vi "F1Machine.vi"() -> ()   [LabVIEW 2011]
doc: "使用该模板构建标准状态机设计模式。各状态执行代码并决定转移状态。将该设计模式与根据用户动作响应而执行代码的用户界面事件处理器模式相比较。同时将该设计模式与队列消息处理模式（各消息处理代码可排队0个或多个新消息）。"
uses:
  F1State.ctl
  API/API DYM.lvlib
panel:
  in  "停止":bool
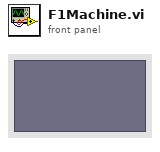
[diagram p1: front panel]
types:
  T1 = typedef "F1State.ctl" = enum16{"Initialize", "Stop", "推送物料", "推料气缸复位", "物件到位检测-光电漫射", "物体属性检测-电涡流", "分拣物体", "不分拣物体", "物件到位检测-电容式接近开关", "气缸机构运动", "气缸机构复位"}
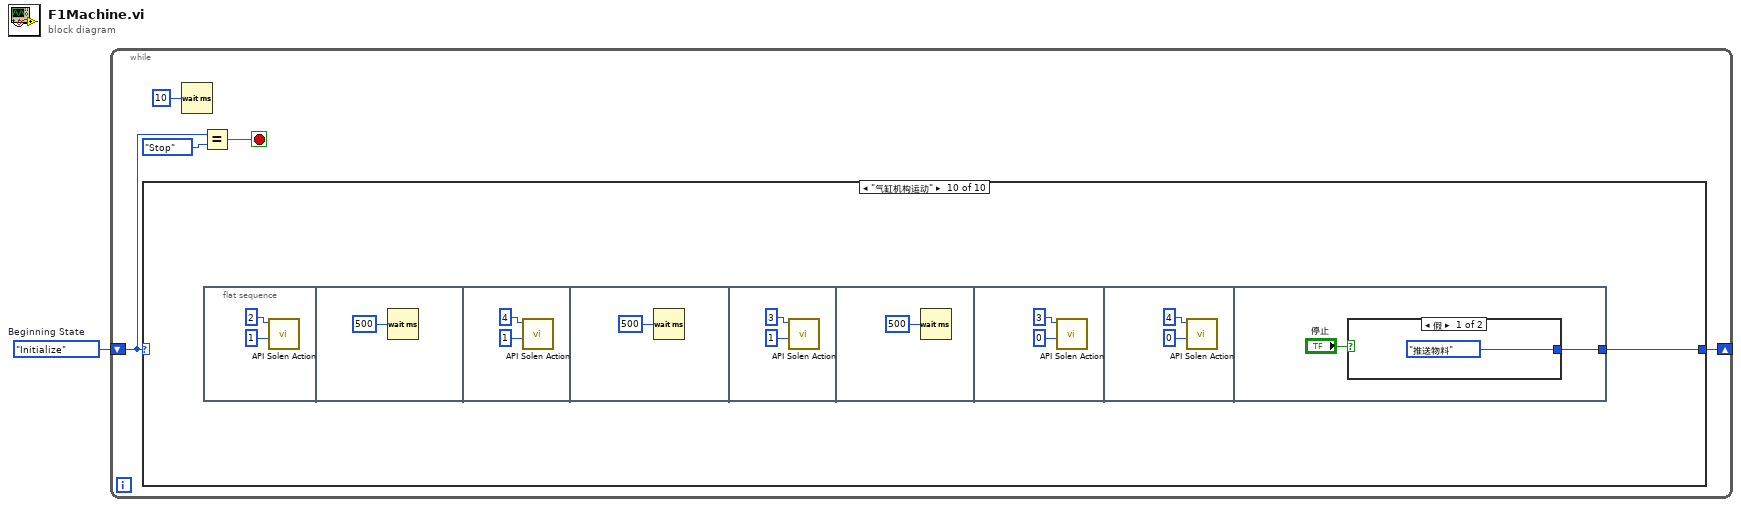
[diagram p0: block diagram]
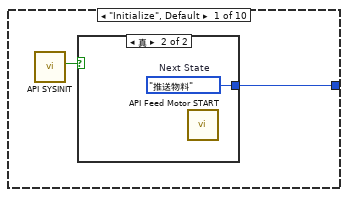
[diagram p2: hidden frame]
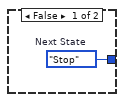
[diagram p3: hidden frame]
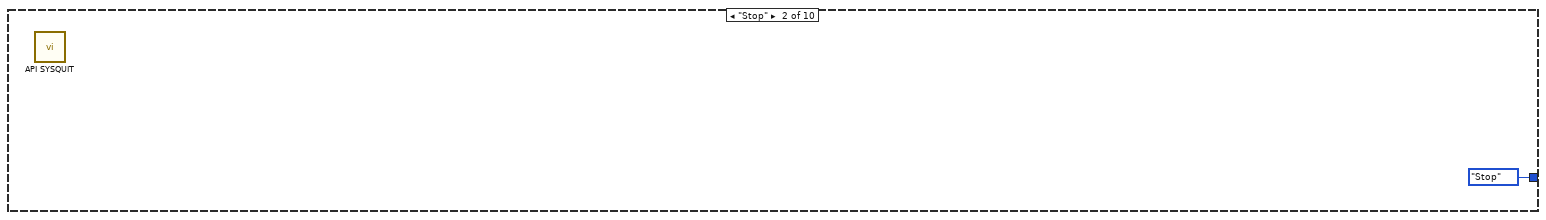
[diagram p4: hidden frame]
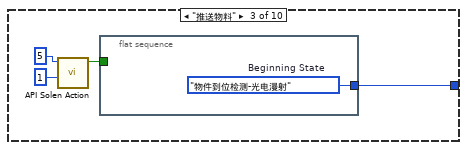
[diagram p5: hidden frame]
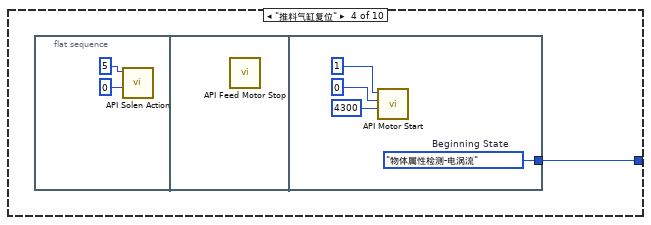
[diagram p6: hidden frame]
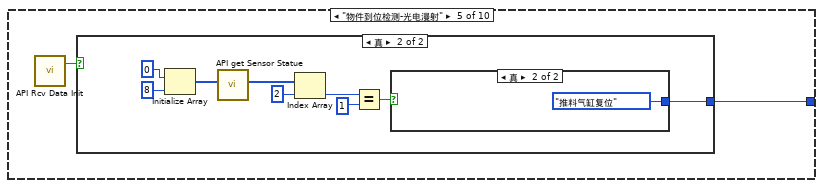
[diagram p7: hidden frame]
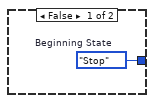
[diagram p8: hidden frame]
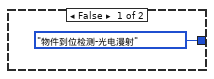
[diagram p9: hidden frame]
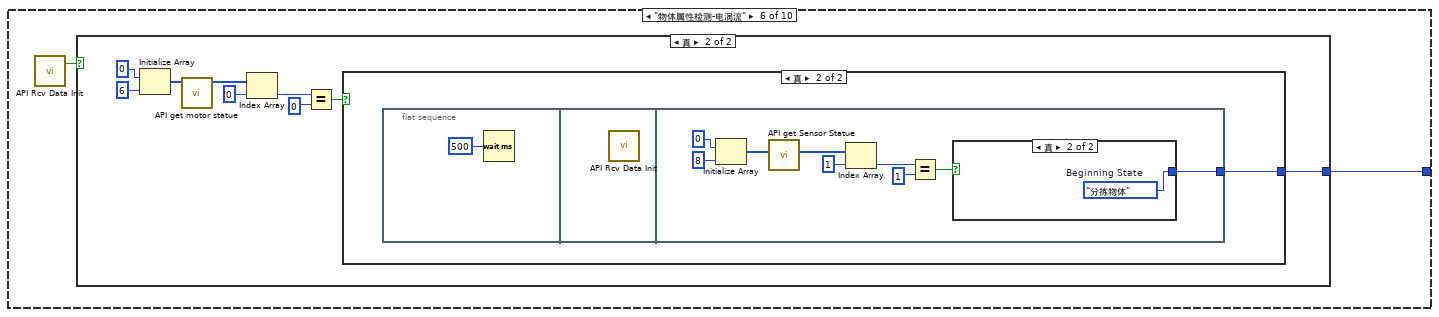
[diagram p10: hidden frame]
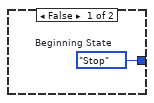
[diagram p11: hidden frame]
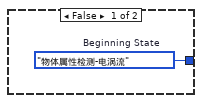
[diagram p12: hidden frame]
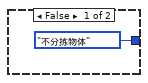
[diagram p13: hidden frame]
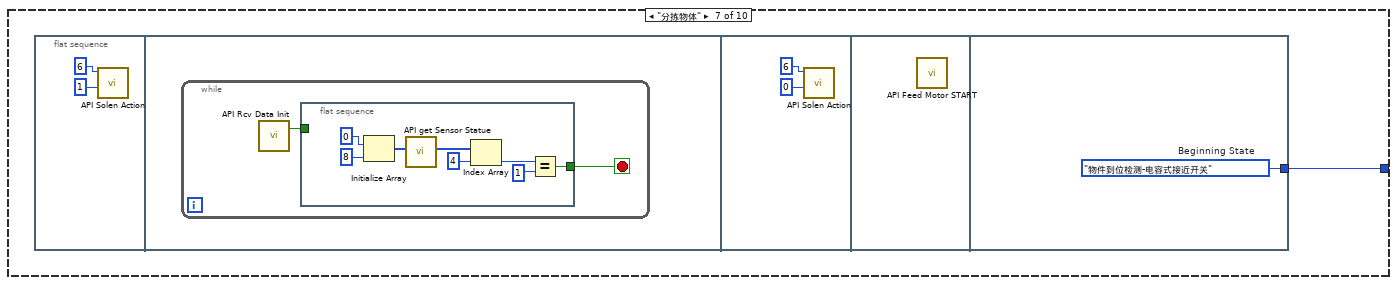
[diagram p14: hidden frame]
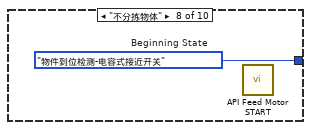
[diagram p15: hidden frame]
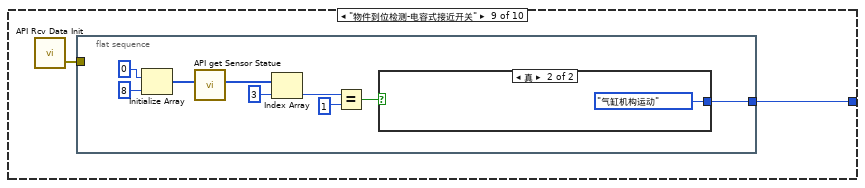
[diagram p16: hidden frame]
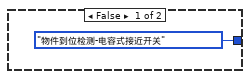
[diagram p17: hidden frame]
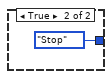
[diagram p18: hidden frame]
diagram:
  w1 = F1State."Initialize"  # Beginning State
  n1 = while {
    shift-right: [w3] -> _
    shift-left: w1 -> [w4]
    stop <- w6 stop-if-true
    n2 = case shown="\"气缸机构运动\"" w4 {
      tunnel: [w7 F1State."Stop" ("Next State") w12 w17 w24 w38 w64 w80 w81 w94] -> w3
      frame "Initialize", Default {
        n3 = call "API SYSINIT.vi"() -> ("SYSINIT return value"=w8:bool)  [unwired: 11 in]
        n4 = case shown="真" w8 {
          tunnel: [w9 w10] -> w7
          frame False {
            w9 = F1State."Stop"  # Next State
          }
          frame True {
            w10 = F1State."推送物料"  # Next State
            n5 = call "API Feed Motor START.vi"() -> ()  [unwired: 11 in, 1 out]
          }
        }
      }
      frame "Stop" {
        n6 = call "API SYSQUIT.vi"() -> ()  [unwired: 12 in]
      }
      frame "推送物料" {
        n7 = call "API Solen Action.vi"("statue"=1, "solenNum"=5) -> ("solenaction return value"=w13:bool)  [unwired: 9 in]
        n8 = flat-sequence {
          tunnel: w13 -> [_]
          tunnel: [w16] -> w12
          frame #0 {
            w16 = F1State."物件到位检测-光电漫射"  # Beginning State
          }
        }
      }
      frame "推料气缸复位" {
        n9 = flat-sequence {
          tunnel: [w20] -> w17
          frame #0 {
            n10 = call "API Solen Action.vi"("statue"=0, "solenNum"=5) -> ()  [unwired: 9 in, 1 out]
          }
          frame #1 {
            n11 = call "API Feed Motor Stop.vi"() -> ()  [unwired: 11 in, 1 out]
          }
          frame #2 {
            w20 = F1State."物体属性检测-电涡流"  # Beginning State
            n12 = call "API Motor Start.vi"("stepNum"=4300, "direction"=0, "motorNum"=1) -> ()  [unwired: 8 in, 1 out]
          }
        }
      }
      frame "物件到位检测-光电漫射" {
        n13 = call "API Rcv Data Init.vi"() -> ("RTV"=w25:bool)  [unwired: 2 in, 1 out]
        n14 = case shown="真" w25 {
          tunnel: [w26 w27] -> w24
          frame False {
            w26 = F1State."Stop"  # Beginning State
          }
          frame True {
            n15 = Initialize Array(0 ("元素"), 8 ("维数大小")) -> (w33:i32[])
            n16 = call "API get Sensor Statue.vi"("array input"=w33) -> ("array output"=w32:i32[])  [unwired: 9 in, 1 out]
            n17 = Index Array(array=w32, index=2 ("索引")) -> (element=w30:i32)
            n18 = Equal?(x=w30, y=1) -> (x = y?=w28:bool)
            n19 = case shown="真" w28 {
              tunnel: [F1State."物件到位检测-光电漫射" ("Beginning State") F1State."推料气缸复位" ("Beginning State")] -> w27
              frame False {
              }
              frame True {
              }
            }
          }
        }
      }
      frame "物体属性检测-电涡流" {
        n20 = call "API Rcv Data Init.vi"() -> ("RTV"=w39:bool)  [unwired: 2 in, 1 out]
        n21 = case shown="真" w39 {
          tunnel: [w40 w41] -> w38
          frame False {
            w40 = F1State."Stop"  # Beginning State
          }
          frame True {
            n22 = Initialize Array(0 ("元素"), 6 ("维数大小")) -> (w47:i32[])
            n23 = call "API get motor statue.vi"("motor statue array input"=w47) -> ("motor statue array output"=w46:i32[])  [unwired: 9 in, 1 out]
            n24 = Index Array(array=w46, index=0 ("索引")) -> (element=w44:i32)
            n25 = Equal?(x=w44, y=0) -> (x = y?=w42:bool)
            n26 = case shown="真" w42 {
              tunnel: [w50 w51] -> w41
              frame False {
                w50 = F1State."物体属性检测-电涡流"  # Beginning State
              }
              frame True {
                n27 = flat-sequence {
                  tunnel: [w53] -> w51
                  frame #0 {
                    n28 = Wait (ms)(milliseconds to wait=u32 500) -> ()  [unwired: 1 out]
                  }
                  frame #1 {
                    n29 = call "API Rcv Data Init.vi"() -> ()  [unwired: 2 in, 2 out]
                  }
                  frame #2 {
                    n30 = Initialize Array(0 ("元素"), 8 ("维数大小")) -> (w59:i32[])
                    n31 = call "API get Sensor Statue.vi"("array input"=w59) -> ("array output"=w58:i32[])  [unwired: 9 in, 1 out]
                    n32 = Index Array(array=w58, index=1 ("索引")) -> (element=w55:i32)
                    n33 = Equal?(x=w55, y=1) -> (x = y?=w54:bool)
                    n34 = case shown="真" w54 {
                      tunnel: [F1State."不分拣物体" ("Beginning State") w63] -> w53
                      frame False {
                      }
                      frame True {
                        w63 = F1State."分拣物体"  # Beginning State
                      }
                    }
                  }
                }
              }
            }
          }
        }
      }
      frame "分拣物体" {
        n35 = flat-sequence {
          tunnel: [w79] -> w64
          frame #0 {
            n36 = call "API Solen Action.vi"("statue"=1, "solenNum"=6) -> ()  [unwired: 9 in, 1 out]
          }
          frame #1 {
            n37 = while {
              stop <- w68 stop-if-true
              n38 = call "API Rcv Data Init.vi"() -> ("RTV"=w67:bool)  [unwired: 2 in, 1 out]
              n39 = flat-sequence {
                tunnel: [w69] -> w68
                tunnel: w67 -> [_]
                frame #0 {
                  n40 = Initialize Array(0 ("元素"), 8 ("维数大小")) -> (w74:i32[])
                  n41 = call "API get Sensor Statue.vi"("array input"=w74) -> ("array output"=w73:i32[])  [unwired: 9 in, 1 out]
                  n42 = Index Array(array=w73, index=4 ("索引")) -> (element=w71:i32)
                  n43 = Equal?(x=w71, y=1) -> (x = y?=w69:bool)
                }
              }
            }
          }
          frame #2 {
            n44 = call "API Solen Action.vi"("statue"=0, "solenNum"=6) -> ()  [unwired: 9 in, 1 out]
          }
          frame #3 {
            n45 = call "API Feed Motor START.vi"() -> ()  [unwired: 11 in, 1 out]
          }
          frame #4 {
            w79 = F1State."物件到位检测-电容式接近开关"  # Beginning State
          }
        }
      }
      frame "不分拣物体" {
        w80 = F1State."物件到位检测-电容式接近开关"  # Beginning State
        n46 = call "API Feed Motor START.vi"() -> ()  [unwired: 11 in, 1 out]
      }
      frame "物件到位检测-电容式接近开关" {
        n47 = call "API Rcv Data Init.vi"() -> ("错误输出"=w82:errorcluster)  [unwired: 2 in, 1 out]
        n48 = flat-sequence {
          tunnel: w82 -> [_]
          tunnel: [w83] -> w81
          frame #0 {
            n49 = Initialize Array(0 ("元素"), 8 ("维数大小")) -> (w89:i32[])
            n50 = call "API get Sensor Statue.vi"("array input"=w89) -> ("array output"=w88:i32[])  [unwired: 9 in, 1 out]
            n51 = Index Array(array=w88, index=3 ("索引")) -> (element=w86:i32)
            n52 = Equal?(x=w86, y=1) -> (x = y?=w84:bool)
            n53 = case shown="真" w84 {
              tunnel: [F1State."物件到位检测-电容式接近开关" ("Beginning State") F1State."气缸机构运动" ("Beginning State")] -> w83
              frame False {
              }
              frame True {
              }
            }
          }
        }
      }
      frame "气缸机构运动" {
        n54 = flat-sequence {
          tunnel: [w108] -> w94
          frame #0 {
            n55 = call "API Solen Action.vi"("statue"=1, "solenNum"=2) -> ()  [unwired: 9 in, 1 out]
          }
          frame #1 {
            n56 = Wait (ms)(milliseconds to wait=u32 500) -> ()  [unwired: 1 out]
          }
          frame #2 {
            n57 = call "API Solen Action.vi"("statue"=1, "solenNum"=4) -> ()  [unwired: 9 in, 1 out]
          }
          frame #3 {
            n58 = Wait (ms)(milliseconds to wait=u32 500) -> ()  [unwired: 1 out]
          }
          frame #4 {
            n59 = call "API Solen Action.vi"("statue"=1, "solenNum"=3) -> ()  [unwired: 9 in, 1 out]
          }
          frame #5 {
            n60 = Wait (ms)(milliseconds to wait=u32 500) -> ()  [unwired: 1 out]
          }
          frame #6 {
            n61 = call "API Solen Action.vi"("statue"=0, "solenNum"=3) -> ()  [unwired: 9 in, 1 out]
          }
          frame #7 {
            n62 = call "API Solen Action.vi"("statue"=0, "solenNum"=4) -> ()  [unwired: 9 in, 1 out]
          }
          frame #8 {
            n63 = case shown="假" "停止" {
              tunnel: [F1State."推送物料" ("States") F1State."Stop" ("States")] -> w108
              frame False {
              }
              frame True {
              }
            }
          }
        }
      }
    }
    n64 = Wait (ms)(milliseconds to wait=u32 10) -> ()  [unwired: 1 out]
    n65 = Equal?(x=w4, y=F1State."Stop" ("States")) -> (x = y?=w6:bool)
  }
